vi "TSPopup.Demo Registration.vi"(8 "error in (no error)":errorcluster, 10 "Tests to Run ref":refnum<vi>, 11 "Signal Settings ref":refnum<vi>) -> (0 "error out":errorcluster)   [LabVIEW 2013]
doc: "VI to hold all the different type registrations for this specific demo.\n\nType Sensitive Popup \nCopyright © 2007, J. David Saunders\nAll rights reserved."
uses:
  TSPopup.Popup Call Parameters.ctl
  TSPopup.Data Type.ctl
panel:
  in  "Show Popup (type only)":T1
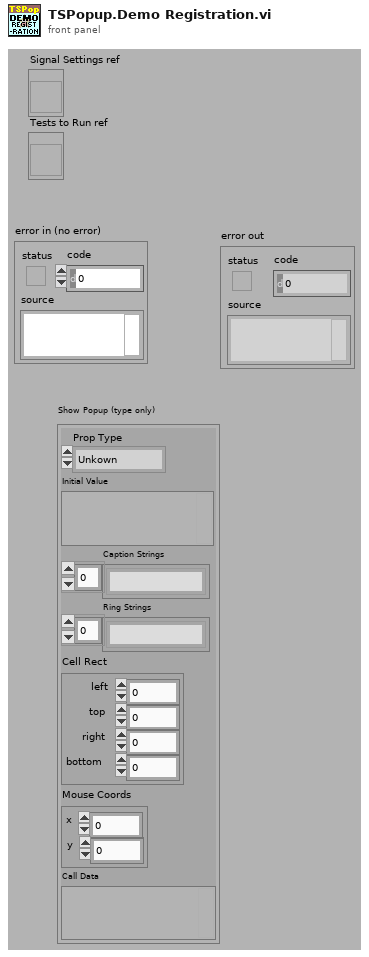
[diagram p1: front panel]
types:
  T1 = typedef "TSPopup.Popup Call Parameters.ctl" = cluster{"Prop Type":T2, "Initial Value":variant, "Caption Strings":string[], "Ring Strings":string[], "Cell Rect":cluster{"left":i16, "top":i16, "right":i16, "bottom":i16}, "Mouse Coords":cluster{"x":i16, "y":i16}, "Call Data":variant}
  T2 = typedef "TSPopup.Data Type.ctl" = enum16{"Unkown", "NO POPUP", "String", "Integer", "Float", "Color", "Boolean", "Ring", "Captioned String", "Captioned Integer", "Button Color", "2 Int Cluster", "4 Int Cluster"}
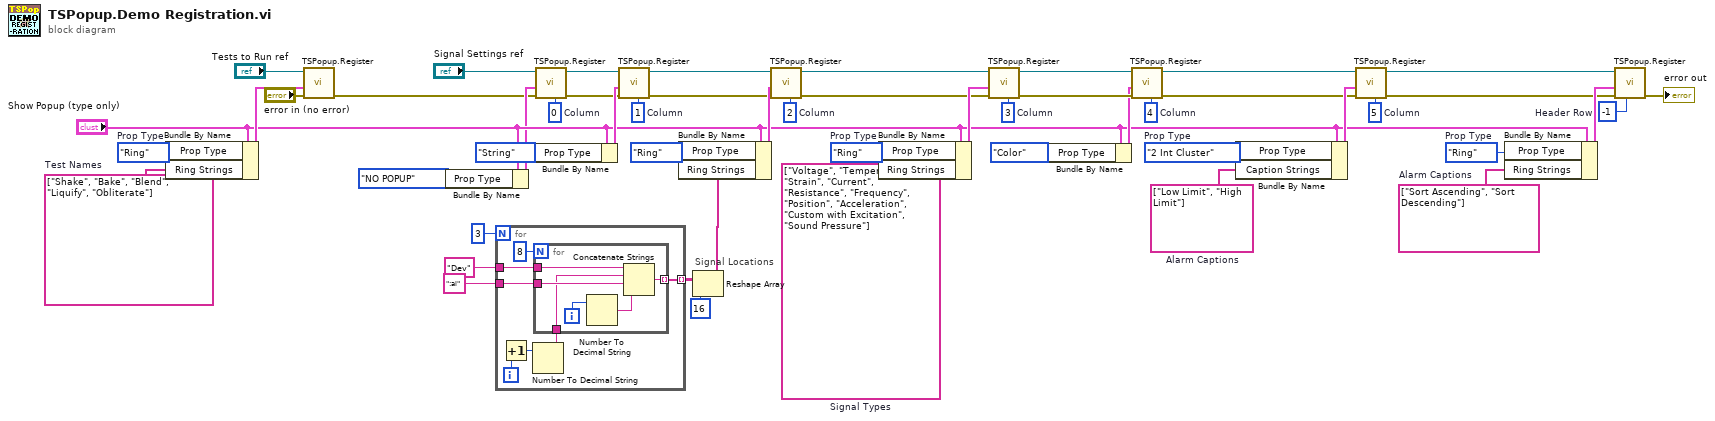
[diagram p0: block diagram]
diagram:
  w9 = 0  # Column
  w1 = -1  # Header Row
  w13 = TSPopup.Data_Type."Ring"  # Prop Type
  w14 = string[] ["Sort Ascending", "Sort Descending"]  # Alarm Captions
  w16 = 5  # Column
  w21 = TSPopup.Data_Type."2 Int Cluster"  # Prop Type
  w27 = 4  # Column
  w34 = 2  # Column
  w35 = 1  # Column
  w39 = 3  # Column
  w42 = TSPopup.Data_Type."Ring"  # Prop Type
  w45 = TSPopup.Data_Type."Ring"  # Prop Type
  w38 = string[] ["Voltage", "Temperature", "Strain", "Current", "Resistance", "Frequency", "Position", "Acceleration", "Custom with Excitation", "Sound Pressure"]  # Signal Types
  w20 = string[] ["Low Limit", "High Limit"]  # Alarm Captions
  w44 = string[] ["Shake", "Bake", "Blend", "Liquify", "Obliterate"]  # Test Names
  # "Signal Locations"
  n1 = Bundle By Name(cluster="Show Popup (type only)", "Prop Type"=w45, "Ring Strings"=w44) -> (w43:T1)
  n2 = call "TSPopup.Register.vi"("error in (no error)"="error in (no error)", "Parameters"=w43, "Ctl Refnum"="Tests to Run ref") -> ("error out"=w2:errorcluster)  [unwired: 7 in, 1 out]
  n3 = Bundle By Name(cluster="Show Popup (type only)", "Prop Type"=TSPopup.Data_Type."NO POPUP") -> (w3:T1)
  n4 = for {
    N: 3 -> [_]
    tunnel: "Dev" -> [w55]
    tunnel: ":ai" -> [w54]
    tunnel: [w52] -> w48 mode=indexing
    i -> [w57]
    n5 = Increment(x=w57) -> (x+1=w56:i32)
    n6 = Number To Decimal String(number=w56) -> (decimal integer string=w53:string)  [unwired: 1 in]
    n7 = for {
      N: 8 -> [_]
      tunnel: w55 -> [w63]
      tunnel: w54 -> [w62]
      tunnel: w53 -> [w61]
      tunnel: [w59] -> w52 mode=indexing
      i -> [w64]
      n8 = Number To Decimal String(number=w64) -> (decimal integer string=w60:string)  [unwired: 1 in]
      n9 = Concatenate Strings(w63, w61, w62, w60) -> (w59:string)
    }
  }
  n10 = Bundle By Name(cluster="Show Popup (type only)", "Prop Type"=TSPopup.Data_Type."String") -> (w36:T1)
  n11 = call "TSPopup.Register.vi"("Col (unwired = all columns)"=w9, "error in (no error)"=w2, "Parameters"=w3, "Ctl Refnum"="Signal Settings ref") -> ("error out"=w7:errorcluster, "dup ref out"=w8:refnum<vi>)  [unwired: 6 in]
  n12 = call "TSPopup.Register.vi"("Col (unwired = all columns)"=w35, "error in (no error)"=w7, "Parameters"=w36, "Ctl Refnum"=w8) -> ("error out"=w30:errorcluster, "dup ref out"=w31:refnum<vi>)  [unwired: 6 in]
  n13 = Reshape Array(w48, 16 ("dimension size")) -> (w29:string[])
  n14 = Bundle By Name(cluster="Show Popup (type only)", "Prop Type"=TSPopup.Data_Type."Ring", "Ring Strings"=w29) -> (w32:T1)
  n15 = call "TSPopup.Register.vi"("Col (unwired = all columns)"=w34, "error in (no error)"=w30, "Parameters"=w32, "Ctl Refnum"=w31) -> ("error out"=w25:errorcluster, "dup ref out"=w26:refnum<vi>)  [unwired: 6 in]
  n16 = Bundle By Name(cluster="Show Popup (type only)", "Prop Type"=w42, "Ring Strings"=w38) -> (w41:T1)
  n17 = call "TSPopup.Register.vi"("Col (unwired = all columns)"=w39, "error in (no error)"=w25, "Parameters"=w41, "Ctl Refnum"=w26) -> ("error out"=w24:errorcluster, "dup ref out"=w23:refnum<vi>)  [unwired: 6 in]
  n18 = Bundle By Name(cluster="Show Popup (type only)", "Prop Type"=TSPopup.Data_Type."Color") -> (w22:T1)
  n19 = call "TSPopup.Register.vi"("Col (unwired = all columns)"=w27, "error in (no error)"=w24, "Parameters"=w22, "Ctl Refnum"=w23) -> ("error out"=w17:errorcluster, "dup ref out"=w18:refnum<vi>)  [unwired: 6 in]
  n20 = Bundle By Name(cluster="Show Popup (type only)", "Prop Type"=w21, "Caption Strings"=w20) -> (w19:T1)
  n21 = call "TSPopup.Register.vi"("Col (unwired = all columns)"=w16, "error in (no error)"=w17, "Parameters"=w19, "Ctl Refnum"=w18) -> ("error out"=w11:errorcluster, "dup ref out"=w10:refnum<vi>)  [unwired: 6 in]
  n22 = Bundle By Name(cluster="Show Popup (type only)", "Prop Type"=w13, "Ring Strings"=w14) -> (w15:T1)
  n23 = call "TSPopup.Register.vi"("Row (unwired = all rows)"=w1, "error in (no error)"=w11, "Parameters"=w15, "Ctl Refnum"=w10) -> ("error out"=→"error out":errorcluster)  [unwired: 6 in, 1 out]
